vi "Lab Panel V4.89.vi"() -> ()   [LabVIEW 2013] (continued)
                    n844 = stacked-sequence {
                      seq-local: [w1534 _] -> [_ w1538]
                      tunnel: w1532 -> [_ w1548]
                      tunnel: w1531 -> [_ w1547]
                      tunnel: w1530 -> [_ w1546]
                      tunnel: w1529 -> [_ w1545]
                      tunnel: w1528 -> [_ w1544]
                      tunnel: [_ w1543] -> w1527
                      tunnel: w1526 -> [_ w1542]
                      tunnel: w1525 -> [_ w1541]
                      tunnel: w1524 -> [_ w1540]
                      tunnel: w1523 -> [w1533 w1539]
                      tunnel: w1522 -> [_ w1537]
                      frame #0 {
                        n845 = Unbundle(w1533) -> ("AMPS"=w1536:dbl)  [unwired: 4 out]
                        n846 = call "Check For Amps on v1.vi"("ID"="LAB04-1", "amps"=w1536) -> ("amps"=w1534:bool)  [unwired: 9 in]
                      }
                      frame #1 {
                        n847 = case shown="True" w1538 {
                          tunnel: w1548 -> [_ w1561]
                          tunnel: w1547 -> [_ w1560]
                          tunnel: w1546 -> [_ w1559]
                          tunnel: w1545 -> [_ w1558]
                          tunnel: w1544 -> [_ w1557]
                          tunnel: [errorcluster {"status"=FALSE, "code"=0, "source"=""} ("error out") w1556] -> w1543
                          tunnel: w1542 -> [_ w1555]
                          tunnel: w1541 -> [_ w1554]
                          tunnel: w1540 -> [_ w1553]
                          tunnel: w1539 -> [_ w1552]
                          tunnel: w1537 -> [_ w1551]
                          frame False {
                            w1549 = FALSE
                            n848 = local write "RUN LAB04-1"(w1549) -> ()
                            n849 = local write "run lab04-1"(w1549) -> ()
                          }
                          frame True {
                            n850 = stacked-sequence {
                              seq-local: [w1562 _ _ _ _] -> [_ w1586 _ _ _]
                              tunnel: w1561 -> [w1567 _ _ _ _]
                              tunnel: w1560 -> [w1563 _ _ _ _]
                              tunnel: w1559 -> [w1577 _ _ _ _]
                              tunnel: w1558 -> [w1570 _ _ _ _]
                              tunnel: w1557 -> [w1565 _ _ _ _]
                              tunnel: [_ w1581 _ _ _] -> w1556
                              tunnel: w1555 -> [_ _ _ w1607 _]
                              tunnel: w1554 -> [_ _ _ w1606 _]
                              tunnel: w1553 -> [_ _ _ w1605 _]
                              tunnel: w1552 -> [_ _ _ _ _]
                              tunnel: w1551 -> [_ _ _ _ w1621]
                              frame #0 {
                                w1564 = "\\"
                                n851 = local read "SET LAB04-1"() -> (w1572:T5)
                                n852 = case shown="\"CYCLE TEST\"" w1577 {
                                tunnel: ["L04-1-CHART TEST-" "L04-1-CYCLE TEST-" "L04-1-T-RISE TEST-"] -> w1573
                                frame "CHART TEST", Default {
                                }
                                frame "CYCLE TEST" {
                                }
                                frame "T-RISE TEST" {
                                }
                                }
                                n853 = Unbundle(w1572) -> ("DESCRIPTION"=w1571:string)  [unwired: 4 out]
                                n854 = Concatenate Strings(w1567, "\\", w1565, w1564, w1563, w1564) -> (w1574:string)
                                n855 = String To Path(string=w1574) -> (path=w1576:path)
                                n856 = Concatenate Strings(w1574, w1573, w1571, "-", w1570, ".tdms") -> (w1562:string)
                                n857 = Create Folder(path (use dialog)=w1576) -> (error out=w1575:errorcluster)  [unwired: 2 in, 2 out]
                                n858 = global write "Global 1.vi" "LAB04-1 FILE"(w1562) -> ()
                                n859 = call <vilib>:"Clear Errors.vi"("error in (no error)"=w1575) -> ()  [unwired: 6 in, 1 out]
                              }
                              frame #1 {
                                (unwired) FALSE
                                n860 = String To Path(string=w1586) -> (path=w1582:path)
                                n861 = TDMS Open(6:FALSE, 10:T20."create or replace" ("operation (0:open)"), 11:w1582) -> (0:w1581:errorcluster, 3:→"TDMS LAB04-1":refnum<k34>)  [unwired: 4 in]
                              }
                              frame #2 {
                                n862 = local read "SET LAB04-1"() -> (w1592:T5)
                                n863 = local read "TDMS LAB04-1"() -> (w1603:refnum<k34>)
                                n864 = Build Array("Testers Name", "Description", "Set Test Cycles", "T-Rise minutes", "T-Rise Deg C") -> (w1593:string[])
                                n865 = Unbundle(w1592) -> ("NAME"=w1591:string, "DESCRIPTION"=w1590:string, "CYCLES"=w1589:dbl, "T-RISE mins"=w1588:dbl, "T-RISE deg C"=w1587:dbl)
                                n866 = Number To Decimal String(number=w1589) -> (decimal integer string=w1602:string)  [unwired: 1 in]
                                n867 = Number To Decimal String(number=w1588) -> (decimal integer string=w1601:string)  [unwired: 1 in]
                                n868 = Number To Decimal String(number=w1587) -> (decimal integer string=w1600:string)  [unwired: 1 in]
                                n869 = Build Array(w1591, w1590, w1602, w1601, w1600) -> (w1599:string[])
                                n870 = TDMS Set Properties(5:w1599, 7:w1593, 11:w1603) -> ()  [unwired: 3 in, 4 out]
                              }
                              frame #3 {
                                n871 = local read "DISP LAB04-1"() -> (w1608:T4)
                                n872 = Concatenate Strings("LAB04-1  ", w1607) -> (w1609:string)
                                n873 = Two Button Dialog(message=w1609, 1:w1605, 2:w1606) -> (T button?=w1611:bool)
                                n874 = case shown="True" w1611 {
                                tunnel: w1608 -> [w1618 w1619]
                                tunnel: [w1618 w1619] -> w1615
                                tunnel: [w1617 w1620] -> w1614
                                tunnel: [w1616 w1620] -> w1613
                                frame False {
                                n875 = Unbundle(w1618) -> ("CYCLE"=w1617:dbl, "MINS"=w1616:dbl)  [unwired: 1 out]
                                }
                                frame True {
                                w1620 = 0.0
                                }
                                }
                                n876 = Bundle(cluster=w1615, "CYCLE"=w1614, "MINS"=w1613, "STATUS"="RUN") -> (w1604:T4)
                                n877 = local write "DISP LAB04-1"(w1604) -> ()
                              }
                              frame #4 {
                                n878 = local read "TEMP START LAB04-1"() -> (w1623:cluster{"TL":dbl, "TN":dbl})
                                n879 = Bundle(cluster=w1623, "TL"=w1621, "TN"=w1621) -> (w1622:cluster{"TL":dbl, "TN":dbl})
                                n880 = local write "TEMP START LAB04-1"(w1622) -> ()
                              }
                            }
                          }
                        }
                      }
                    }
                  }
                }
              }
              event "RUN LAB04-2": Value Change {
                n881 = event-data() -> ("NewVal"=w1628:bool)  [unwired: 1 in, 5 out]
                n882 = local write "run lab04-2"(w1628) -> ()
                n883 = case shown="True" w1628 {
                  tunnel: w1634 -> [_ w1672]
                  tunnel: w1633 -> [_ w1671]
                  tunnel: w1631 -> [w1636 w1670]
                  tunnel: w1632 -> [_ w1669]
                  tunnel: w1630 -> [_ w1668]
                  tunnel: [w1635 w1667] -> w1629
                  tunnel: w1627 -> [_ w1666]
                  tunnel: w1626 -> [_ w1665]
                  tunnel: w1625 -> [_ w1664]
                  tunnel: w1624 -> [_ w1662]
                  frame False {
                    # "stop test"
                    n884 = stacked-sequence {
                      tunnel: w1636 -> [w1645 _]
                      tunnel: [w1637 _] -> w1635
                      frame #0 {
                        n885 = local read "DISP LAB04-2"() -> (w1644:T4)
                        n886 = Unbundle(w1644) -> ("CYCLE"=w1642:dbl, "MINS"=w1643:dbl)  [unwired: 1 out]
                        n887 = case shown="\"CYCLE TEST\"" w1645 {
                          tunnel: w1643 -> [_ _ w1652]
                          tunnel: w1642 -> [w1650 w1651 _]
                          tunnel: [w1650 w1651 w1652] -> w1641
                          frame "CHART TEST", Default {
                          }
                          frame "CYCLE TEST" {
                          }
                          frame "T-RISE TEST" {
                          }
                        }
                        n888 = local read "TDMS LAB04-2"() -> (w1649:refnum<k34>)
                        n889 = Build Array("STOPPED") -> (w1646:string[])
                        n890 = Build Array(w1641) -> (w1640:dbl[])
                        n891 = TDMS Write(0:w1649, 5:"TEST RESULT", 7:w1646, 9:w1640) -> (4:w1638:refnum<k34>, 15:w1639:errorcluster)  [unwired: 2 in, 2 out]
                        n892 = TDMS Close(8:w1639, 11:w1638) -> (0:w1637:errorcluster)  [unwired: 1 out]
                      }
                      frame #1 {
                        n893 = local read "DISP LAB04-2"() -> (w1656:T4)
                        n894 = stacked-sequence {
                          tunnel: "LAB04-2" -> [w1658 w1660]
                          frame #0 {
                            n895 = call "sub vi - defrag tdms v1.vi"("panel id"=w1658) -> ("error out"=w1657:errorcluster)  [unwired: 10 in]
                            n896 = local write "data file error"(w1657) -> ()
                          }
                          frame #1 {
                            n897 = call "Save data file (stop) v3.vi"("panel id"=w1660) -> ("network file save error"=w1659:errorcluster)  [unwired: 9 in, 1 out]
                            n898 = local write "RESULT LAB04-2"(FALSE) -> ()
                            n899 = local write "data file error"(w1659) -> ()
                          }
                        }
                        n900 = Bundle(cluster=w1656, "STATUS"="STOP") -> (w1654:T4)  [unwired: 2 in]
                        n901 = local write "DISP LAB04-2"(w1654) -> ()
                      }
                    }
                  }
                  frame True {
                    n902 = local read "SIG LAB04-2"() -> (w1663:T2)
                    n903 = stacked-sequence {
                      seq-local: [w1674 _] -> [_ w1678]
                      tunnel: w1672 -> [_ w1688]
                      tunnel: w1671 -> [_ w1687]
                      tunnel: w1670 -> [_ w1686]
                      tunnel: w1669 -> [_ w1685]
                      tunnel: w1668 -> [_ w1684]
                      tunnel: [_ w1683] -> w1667
                      tunnel: w1666 -> [_ w1682]
                      tunnel: w1665 -> [_ w1681]
                      tunnel: w1664 -> [_ w1680]
                      tunnel: w1663 -> [w1673 w1679]
                      tunnel: w1662 -> [_ w1677]
                      frame #0 {
                        n904 = Unbundle(w1673) -> ("AMPS"=w1676:dbl)  [unwired: 4 out]
                        n905 = call "Check For Amps on v1.vi"("ID"="LAB04-2", "amps"=w1676) -> ("amps"=w1674:bool)  [unwired: 9 in]
                      }
                      frame #1 {
                        n906 = case shown="True" w1678 {
                          tunnel: w1688 -> [_ w1701]
                          tunnel: w1687 -> [_ w1700]
                          tunnel: w1686 -> [_ w1699]
                          tunnel: w1685 -> [_ w1698]
                          tunnel: w1684 -> [_ w1697]
                          tunnel: [errorcluster {"status"=FALSE, "code"=0, "source"=""} ("error out") w1696] -> w1683
                          tunnel: w1682 -> [_ w1695]
                          tunnel: w1681 -> [_ w1694]
                          tunnel: w1680 -> [_ w1693]
                          tunnel: w1679 -> [_ w1692]
                          tunnel: w1677 -> [_ w1691]
                          frame False {
                            w1689 = FALSE
                            n907 = local write "RUN LAB04-2"(w1689) -> ()
                            n908 = local write "run lab04-2"(w1689) -> ()
                          }
                          frame True {
                            n909 = stacked-sequence {
                              seq-local: [w1702 _ _ _ _] -> [_ w1726 _ _ _]
                              tunnel: w1701 -> [w1707 _ _ _ _]
                              tunnel: w1700 -> [w1703 _ _ _ _]
                              tunnel: w1699 -> [w1717 _ _ _ _]
                              tunnel: w1698 -> [w1710 _ _ _ _]
                              tunnel: w1697 -> [w1705 _ _ _ _]
                              tunnel: [_ w1721 _ _ _] -> w1696
                              tunnel: w1695 -> [_ _ _ w1747 _]
                              tunnel: w1694 -> [_ _ _ w1746 _]
                              tunnel: w1693 -> [_ _ _ w1745 _]
                              tunnel: w1692 -> [_ _ _ _ _]
                              tunnel: w1691 -> [_ _ _ _ w1761]
                              frame #0 {
                                w1704 = "\\"
                                n910 = local read "SET LAB04-2"() -> (w1712:T5)
                                n911 = case shown="\"CHART TEST\", Default" w1717 {
                                tunnel: ["L04-2-CHART TEST-" "L04-2-CYCLE TEST-" "L04-2-T-RISE TEST-"] -> w1713
                                frame "CHART TEST", Default {
                                }
                                frame "CYCLE TEST" {
                                }
                                frame "T-RISE TEST" {
                                }
                                }
                                n912 = Unbundle(w1712) -> ("DESCRIPTION"=w1711:string)  [unwired: 4 out]
                                n913 = Concatenate Strings(w1707, "\\", w1705, w1704, w1703, w1704) -> (w1714:string)
                                n914 = String To Path(string=w1714) -> (path=w1716:path)
                                n915 = Concatenate Strings(w1714, w1713, w1711, "-", w1710, ".tdms") -> (w1702:string)
                                n916 = Create Folder(path (use dialog)=w1716) -> (error out=w1715:errorcluster)  [unwired: 2 in, 2 out]
                                n917 = global write "Global 1.vi" "LAB04-2 FILE"(w1702) -> ()
                                n918 = call <vilib>:"Clear Errors.vi"("error in (no error)"=w1715) -> ()  [unwired: 6 in, 1 out]
                              }
                              frame #1 {
                                (unwired) FALSE
                                n919 = String To Path(string=w1726) -> (path=w1722:path)
                                n920 = TDMS Open(6:FALSE, 10:T20."create or replace" ("operation (0:open)"), 11:w1722) -> (0:w1721:errorcluster, 3:→"TDMS LAB04-2":refnum<k34>)  [unwired: 4 in]
                              }
                              frame #2 {
                                n921 = local read "SET LAB04-2"() -> (w1732:T5)
                                n922 = local read "TDMS LAB04-2"() -> (w1743:refnum<k34>)
                                n923 = Build Array("Testers Name", "Description", "Set Test Cycles", "T-Rise minutes", "T-Rise Deg C") -> (w1733:string[])
                                n924 = Unbundle(w1732) -> ("NAME"=w1731:string, "DESCRIPTION"=w1730:string, "CYCLES"=w1729:dbl, "T-RISE mins"=w1728:dbl, "T-RISE deg C"=w1727:dbl)
                                n925 = Number To Decimal String(number=w1729) -> (decimal integer string=w1742:string)  [unwired: 1 in]
                                n926 = Number To Decimal String(number=w1728) -> (decimal integer string=w1741:string)  [unwired: 1 in]
                                n927 = Number To Decimal String(number=w1727) -> (decimal integer string=w1740:string)  [unwired: 1 in]
                                n928 = Build Array(w1731, w1730, w1742, w1741, w1740) -> (w1739:string[])
                                n929 = TDMS Set Properties(5:w1739, 7:w1733, 11:w1743) -> ()  [unwired: 3 in, 4 out]
                              }
                              frame #3 {
                                n930 = local read "DISP LAB04-2"() -> (w1748:T4)
                                n931 = Concatenate Strings("LAB04-2 ", w1747) -> (w1749:string)
                                n932 = Two Button Dialog(message=w1749, 1:w1745, 2:w1746) -> (T button?=w1751:bool)
                                n933 = case shown="True" w1751 {
                                tunnel: w1748 -> [w1758 w1759]
                                tunnel: [w1758 w1759] -> w1755
                                tunnel: [w1757 w1760] -> w1754
                                tunnel: [w1756 w1760] -> w1753
                                frame False {
                                n934 = Unbundle(w1758) -> ("CYCLE"=w1757:dbl, "MINS"=w1756:dbl)  [unwired: 1 out]
                                }
                                frame True {
                                w1760 = 0.0
                                }
                                }
                                n935 = Bundle(cluster=w1755, "CYCLE"=w1754, "MINS"=w1753, "STATUS"="RUN") -> (w1744:T4)
                                n936 = local write "DISP LAB04-2"(w1744) -> ()
                              }
                              frame #4 {
                                n937 = local read "TEMP START LAB04-2"() -> (w1763:cluster{"TL":dbl, "TN":dbl})
                                n938 = Bundle(cluster=w1763, "TL"=w1761, "TN"=w1761) -> (w1762:cluster{"TL":dbl, "TN":dbl})
                                n939 = local write "TEMP START LAB04-2"(w1762) -> ()
                              }
                            }
                          }
                        }
                      }
                    }
                  }
                }
              }
              event "RUN LAB05-1": Value Change {
                n940 = event-data() -> ("NewVal"=w1768:bool)  [unwired: 1 in, 5 out]
                n941 = local write "run lab05-1"(w1768) -> ()
                n942 = case shown="True" w1768 {
                  tunnel: w1774 -> [_ w1812]
                  tunnel: w1773 -> [_ w1811]
                  tunnel: w1771 -> [w1776 w1810]
                  tunnel: w1772 -> [_ w1809]
                  tunnel: w1770 -> [_ w1808]
                  tunnel: [w1775 w1807] -> w1769
                  tunnel: w1767 -> [_ w1806]
                  tunnel: w1766 -> [_ w1805]
                  tunnel: w1765 -> [_ w1804]
                  tunnel: w1764 -> [_ w1802]
                  frame False {
                    # "stop test"
                    n943 = stacked-sequence {
                      tunnel: w1776 -> [w1785 _]
                      tunnel: [w1777 _] -> w1775
                      frame #0 {
                        n944 = local read "DISP LAB05-1"() -> (w1784:T4)
                        n945 = Unbundle(w1784) -> ("CYCLE"=w1782:dbl, "MINS"=w1783:dbl)  [unwired: 1 out]
                        n946 = case shown="\"CYCLE TEST\"" w1785 {
                          tunnel: w1783 -> [_ _ w1792]
                          tunnel: w1782 -> [w1790 w1791 _]
                          tunnel: [w1790 w1791 w1792] -> w1781
                          frame "CHART TEST", Default {
                          }
                          frame "CYCLE TEST" {
                          }
                          frame "T-RISE TEST" {
                          }
                        }
                        n947 = local read "TDMS LAB05-1"() -> (w1789:refnum<k34>)
                        n948 = Build Array("STOPPED") -> (w1786:string[])
                        n949 = Build Array(w1781) -> (w1780:dbl[])
                        n950 = TDMS Write(0:w1789, 5:"TEST RESULT", 7:w1786, 9:w1780) -> (4:w1778:refnum<k34>, 15:w1779:errorcluster)  [unwired: 2 in, 2 out]
                        n951 = TDMS Close(8:w1779, 11:w1778) -> (0:w1777:errorcluster)  [unwired: 1 out]
                      }
                      frame #1 {
                        n952 = local read "DISP LAB05-1"() -> (w1796:T4)
                        n953 = stacked-sequence {
                          tunnel: "LAB05-1" -> [w1798 w1800]
                          frame #0 {
                            n954 = call "sub vi - defrag tdms v1.vi"("panel id"=w1798) -> ("error out"=w1797:errorcluster)  [unwired: 10 in]
                            n955 = local write "data file error"(w1797) -> ()
                          }
                          frame #1 {
                            n956 = call "Save data file (stop) v3.vi"("panel id"=w1800) -> ("network file save error"=w1799:errorcluster)  [unwired: 9 in, 1 out]
                            n957 = local write "RESULT LAB05-1"(FALSE) -> ()
                            n958 = local write "data file error"(w1799) -> ()
                          }
                        }
                        n959 = Bundle(cluster=w1796, "STATUS"="STOP") -> (w1794:T4)  [unwired: 2 in]
                        n960 = local write "DISP LAB05-1"(w1794) -> ()
                      }
                    }
                  }
                  frame True {
                    n961 = local read "SIG LAB05-1"() -> (w1803:T2)
                    n962 = stacked-sequence {
                      seq-local: [w1814 _] -> [_ w1818]
                      tunnel: w1812 -> [_ w1828]
                      tunnel: w1811 -> [_ w1827]
                      tunnel: w1810 -> [_ w1826]
                      tunnel: w1809 -> [_ w1825]
                      tunnel: w1808 -> [_ w1824]
                      tunnel: [_ w1823] -> w1807
                      tunnel: w1806 -> [_ w1822]
                      tunnel: w1805 -> [_ w1821]
                      tunnel: w1804 -> [_ w1820]
                      tunnel: w1803 -> [w1813 w1819]
                      tunnel: w1802 -> [_ w1817]
                      frame #0 {
                        n963 = Unbundle(w1813) -> ("AMPS"=w1816:dbl)  [unwired: 4 out]
                        n964 = call "Check For Amps on v1.vi"("ID"="LAB05-1", "amps"=w1816) -> ("amps"=w1814:bool)  [unwired: 9 in]
                      }
                      frame #1 {
                        n965 = case shown="True" w1818 {
                          tunnel: w1828 -> [_ w1841]
                          tunnel: w1827 -> [_ w1840]
                          tunnel: w1826 -> [_ w1839]
                          tunnel: w1825 -> [_ w1838]
                          tunnel: w1824 -> [_ w1837]
                          tunnel: [errorcluster {"status"=FALSE, "code"=0, "source"=""} ("error out") w1836] -> w1823
                          tunnel: w1822 -> [_ w1835]
                          tunnel: w1821 -> [_ w1834]
                          tunnel: w1820 -> [_ w1833]
                          tunnel: w1819 -> [_ w1832]
                          tunnel: w1817 -> [_ w1831]
                          frame False {
                            w1829 = FALSE
                            n966 = local write "RUN LAB05-1"(w1829) -> ()
                            n967 = local write "run lab05-1"(w1829) -> ()
                          }
                          frame True {
                            n968 = stacked-sequence {
                              seq-local: [w1842 _ _ _ _] -> [_ w1866 _ _ _]
                              tunnel: w1841 -> [w1847 _ _ _ _]
                              tunnel: w1840 -> [w1843 _ _ _ _]
                              tunnel: w1839 -> [w1857 _ _ _ _]
                              tunnel: w1838 -> [w1850 _ _ _ _]
                              tunnel: w1837 -> [w1845 _ _ _ _]
                              tunnel: [_ w1861 _ _ _] -> w1836
                              tunnel: w1835 -> [_ _ _ w1886 _]
                              tunnel: w1834 -> [_ _ _ w1885 _]
                              tunnel: w1833 -> [_ _ _ w1884 _]
                              tunnel: w1832 -> [_ _ _ _ _]
                              tunnel: w1831 -> [_ _ _ _ w1901]
                              frame #0 {
                                w1844 = "\\"
                                n969 = local read "SET LAB05-1"() -> (w1852:T5)
                                n970 = case shown="\"CYCLE TEST\"" w1857 {
                                tunnel: ["L05-1-CHART TEST-" "L05-1-CYCLE TEST-" "L05-1-T-RISE TEST-"] -> w1853
                                frame "CHART TEST", Default {
                                }
                                frame "CYCLE TEST" {
                                }
                                frame "T-RISE TEST" {
                                }
                                }
                                n971 = Unbundle(w1852) -> ("DESCRIPTION"=w1851:string)  [unwired: 4 out]
                                n972 = Concatenate Strings(w1847, "\\", w1845, w1844, w1843, w1844) -> (w1854:string)
                                n973 = String To Path(string=w1854) -> (path=w1856:path)
                                n974 = Concatenate Strings(w1854, w1853, w1851, "-", w1850, ".tdms") -> (w1842:string)
                                n975 = Create Folder(path (use dialog)=w1856) -> (error out=w1855:errorcluster)  [unwired: 2 in, 2 out]
                                n976 = global write "Global 1.vi" "LAB05-1 FILE"(w1842) -> ()
                                n977 = call <vilib>:"Clear Errors.vi"("error in (no error)"=w1855) -> ()  [unwired: 6 in, 1 out]
                              }
                              frame #1 {
                                (unwired) FALSE
                                n978 = String To Path(string=w1866) -> (path=w1862:path)
                                n979 = TDMS Open(6:FALSE, 10:T20."create or replace" ("operation (0:open)"), 11:w1862) -> (0:w1861:errorcluster, 3:→"TDMS LAB05-1":refnum<k34>)  [unwired: 4 in]
                              }
                              frame #2 {
                                n980 = local read "SET LAB05-1"() -> (w1872:T5)
                                n981 = local read "TDMS LAB05-1"() -> (w1883:refnum<k34>)
                                n982 = Build Array("Testers Name", "Description", "Set Test Cycles", "T-Rise minutes", "T-Rise Deg C") -> (w1873:string[])
                                n983 = Unbundle(w1872) -> ("NAME"=w1871:string, "DESCRIPTION"=w1870:string, "CYCLES"=w1869:dbl, "T-RISE mins"=w1868:dbl, "T-RISE deg C"=w1867:dbl)
                                n984 = Number To Decimal String(number=w1869) -> (decimal integer string=w1882:string)  [unwired: 1 in]
                                n985 = Number To Decimal String(number=w1868) -> (decimal integer string=w1881:string)  [unwired: 1 in]
                                n986 = Number To Decimal String(number=w1867) -> (decimal integer string=w1880:string)  [unwired: 1 in]
                                n987 = Build Array(w1871, w1870, w1882, w1881, w1880) -> (w1879:string[])
                                n988 = TDMS Set Properties(5:w1879, 7:w1873, 11:w1883) -> ()  [unwired: 3 in, 4 out]
                              }
                              frame #3 {
                                n989 = local read "DISP LAB05-1"() -> (w1888:T4)
                                n990 = Concatenate Strings("LAB05-1  ", w1886) -> (w1889:string)
                                n991 = Two Button Dialog(message=w1889, 1:w1884, 2:w1885) -> (T button?=w1891:bool)
                                n992 = case shown="True" w1891 {
                                tunnel: w1888 -> [w1898 w1899]
                                tunnel: [w1898 w1899] -> w1895
                                tunnel: [w1897 w1900] -> w1894
                                tunnel: [w1896 w1900] -> w1893
                                frame False {
                                n993 = Unbundle(w1898) -> ("CYCLE"=w1897:dbl, "MINS"=w1896:dbl)  [unwired: 1 out]
                                }
                                frame True {
                                w1900 = 0.0
                                }
                                }
                                n994 = Bundle(cluster=w1895, "CYCLE"=w1894, "MINS"=w1893, "STATUS"="RUN") -> (w1887:T4)
                                n995 = local write "DISP LAB05-1"(w1887) -> ()
                              }
                              frame #4 {
                                n996 = local read "TEMP START LAB05-1"() -> (w1903:cluster{"TL":dbl, "TN":dbl})
                                n997 = Bundle(cluster=w1903, "TL"=w1901, "TN"=w1901) -> (w1902:cluster{"TL":dbl, "TN":dbl})
                                n998 = local write "TEMP START LAB05-1"(w1902) -> ()
                              }
                            }
                          }
                        }
                      }
                    }
                  }
                }
              }
              event "RUN LAB05-2": Value Change {
                n999 = event-data() -> ("NewVal"=w1909:bool)  [unwired: 1 in, 5 out]
                n1000 = local read "SIG LAB05-2"() -> (w1905:T2)
                n1001 = case shown="True" w1909 {
                  tunnel: w1915 -> [_ w1953]
                  tunnel: w1914 -> [_ w1952]
                  tunnel: w1912 -> [w1917 w1951]
                  tunnel: w1913 -> [_ w1950]
                  tunnel: w1911 -> [_ w1949]
                  tunnel: [w1916 w1948] -> w1910
                  tunnel: w1908 -> [_ w1947]
                  tunnel: w1907 -> [_ w1946]
                  tunnel: w1906 -> [_ w1945]
                  tunnel: w1905 -> [_ w1944]
                  tunnel: w1904 -> [_ w1943]
                  frame False {
                    # "stop test"
                    n1002 = stacked-sequence {
                      tunnel: w1917 -> [w1926 _]
                      tunnel: [w1918 _] -> w1916
                      frame #0 {
                        n1003 = local read "DISP LAB05-2"() -> (w1925:T4)
                        n1004 = Unbundle(w1925) -> ("CYCLE"=w1923:dbl, "MINS"=w1924:dbl)  [unwired: 1 out]
                        n1005 = case shown="\"CYCLE TEST\"" w1926 {
                          tunnel: w1924 -> [_ _ w1933]
                          tunnel: w1923 -> [w1931 w1932 _]
                          tunnel: [w1931 w1932 w1933] -> w1922
                          frame "CHART TEST", Default {
                          }
                          frame "CYCLE TEST" {
                          }
                          frame "T-RISE TEST" {
                          }
                        }
                        n1006 = local read "TDMS LAB05-2"() -> (w1930:refnum<k34>)
                        n1007 = Build Array("STOPPED") -> (w1927:string[])
                        n1008 = Build Array(w1922) -> (w1921:dbl[])
                        n1009 = TDMS Write(0:w1930, 5:"TEST RESULT", 7:w1927, 9:w1921) -> (4:w1919:refnum<k34>, 15:w1920:errorcluster)  [unwired: 2 in, 2 out]
                        n1010 = TDMS Close(8:w1920, 11:w1919) -> (0:w1918:errorcluster)  [unwired: 1 out]
                      }
                      frame #1 {
                        n1011 = local read "DISP LAB05-2"() -> (w1937:T4)
                        n1012 = stacked-sequence {
                          tunnel: "LAB05-2" -> [w1939 w1941]
                          frame #0 {
                            n1013 = call "sub vi - defrag tdms v1.vi"("panel id"=w1939) -> ("error out"=w1938:errorcluster)  [unwired: 10 in]
                            n1014 = local write "data file error"(w1938) -> ()
                          }
                          frame #1 {
                            n1015 = local write "RESULT LAB05-2"(FALSE) -> ()
                            n1016 = call "Save data file (stop) v3.vi"("panel id"=w1941) -> ("network file save error"=w1940:errorcluster)  [unwired: 9 in, 1 out]
                            n1017 = local write "data file error"(w1940) -> ()
                          }
                        }
                        n1018 = Bundle(cluster=w1937, "STATUS"="STOP") -> (w1935:T4)  [unwired: 2 in]
                        n1019 = local write "DISP LAB05-2"(w1935) -> ()
                      }
                    }
                  }
                  frame True {
                    n1020 = stacked-sequence {
                      seq-local: [w1955 _] -> [_ w1959]
                      tunnel: w1953 -> [_ w1969]
                      tunnel: w1952 -> [_ w1968]
                      tunnel: w1951 -> [_ w1967]
                      tunnel: w1950 -> [_ w1966]
                      tunnel: w1949 -> [_ w1965]
                      tunnel: [_ w1964] -> w1948
                      tunnel: w1947 -> [_ w1963]
                      tunnel: w1946 -> [_ w1962]
                      tunnel: w1945 -> [_ w1961]
                      tunnel: w1944 -> [w1954 w1960]
                      tunnel: w1943 -> [_ w1958]
                      frame #0 {
                        n1021 = Unbundle(w1954) -> ("AMPS"=w1957:dbl)  [unwired: 4 out]
                        n1022 = call "Check For Amps on v1.vi"("ID"="LAB05-2", "amps"=w1957) -> ("amps"=w1955:bool)  [unwired: 9 in]
                      }
                      frame #1 {
                        n1023 = case shown="True" w1959 {
                          tunnel: w1969 -> [_ w1982]
                          tunnel: w1968 -> [_ w1981]
                          tunnel: w1967 -> [_ w1980]
                          tunnel: w1966 -> [_ w1979]
                          tunnel: w1965 -> [_ w1978]
                          tunnel: [errorcluster {"status"=FALSE, "code"=0, "source"=""} ("error out") w1977] -> w1964
                          tunnel: w1963 -> [_ w1976]
                          tunnel: w1962 -> [_ w1975]
                          tunnel: w1961 -> [_ w1974]
                          tunnel: w1960 -> [_ w1973]
                          tunnel: w1958 -> [_ w1972]
                          frame False {
                            w1970 = FALSE
                            n1024 = local write "RUN LAB05-2"(w1970) -> ()
                            n1025 = local write "run lab05-2"(w1970) -> ()
                          }
                          frame True {
                            n1026 = stacked-sequence {
                              seq-local: [w1983 _ _ _ _] -> [_ w2007 _ _ _]
                              tunnel: w1982 -> [w1988 _ _ _ _]
                              tunnel: w1981 -> [w1984 _ _ _ _]
                              tunnel: w1980 -> [w1998 _ _ _ _]
                              tunnel: w1979 -> [w1991 _ _ _ _]
                              tunnel: w1978 -> [w1986 _ _ _ _]
                              tunnel: [_ w2002 _ _ _] -> w1977
                              tunnel: w1976 -> [_ _ _ w2027 _]
                              tunnel: w1975 -> [_ _ _ w2026 _]
                              tunnel: w1974 -> [_ _ _ w2025 _]
                              tunnel: w1973 -> [_ _ _ _ _]
                              tunnel: w1972 -> [_ _ _ _ w2042]
                              frame #0 {
                                w1985 = "\\"
                                n1027 = local read "SET LAB05-2"() -> (w1993:T5)
                                n1028 = case shown="\"CYCLE TEST\"" w1998 {
                                tunnel: ["L05-2-CHART TEST-" "L05-2-CYCLE TEST-" "L05-2-T-RISE TEST-"] -> w1994
                                frame "CHART TEST", Default {
                                }
                                frame "CYCLE TEST" {
                                }
                                frame "T-RISE TEST" {
                                }
                                }
                                n1029 = Unbundle(w1993) -> ("DESCRIPTION"=w1992:string)  [unwired: 4 out]
                                n1030 = Concatenate Strings(w1988, "\\", w1986, w1985, w1984, w1985) -> (w1995:string)
                                n1031 = String To Path(string=w1995) -> (path=w1997:path)
                                n1032 = Concatenate Strings(w1995, w1994, w1992, "-", w1991, ".tdms") -> (w1983:string)
                                n1033 = Create Folder(path (use dialog)=w1997) -> (error out=w1996:errorcluster)  [unwired: 2 in, 2 out]
                                n1034 = global write "Global 1.vi" "LAB05-2 FILE"(w1983) -> ()
                                n1035 = call <vilib>:"Clear Errors.vi"("error in (no error)"=w1996) -> ()  [unwired: 6 in, 1 out]
                              }
                              frame #1 {
                                (unwired) FALSE
                                n1036 = String To Path(string=w2007) -> (path=w2003:path)
                                n1037 = TDMS Open(6:FALSE, 10:T20."create or replace" ("operation (0:open)"), 11:w2003) -> (0:w2002:errorcluster, 3:→"TDMS LAB05-2":refnum<k34>)  [unwired: 4 in]
                              }
                              frame #2 {
                                n1038 = local read "SET LAB05-2"() -> (w2013:T5)
                                n1039 = local read "TDMS LAB05-2"() -> (w2024:refnum<k34>)
                                n1040 = Build Array("Testers Name", "Description", "Set Test Cycles", "T-Rise minutes", "T-Rise Deg C") -> (w2014:string[])
                                n1041 = Unbundle(w2013) -> ("NAME"=w2012:string, "DESCRIPTION"=w2011:string, "CYCLES"=w2010:dbl, "T-RISE mins"=w2009:dbl, "T-RISE deg C"=w2008:dbl)
                                n1042 = Number To Decimal String(number=w2010) -> (decimal integer string=w2023:string)  [unwired: 1 in]
                                n1043 = Number To Decimal String(number=w2009) -> (decimal integer string=w2022:string)  [unwired: 1 in]
                                n1044 = Number To Decimal String(number=w2008) -> (decimal integer string=w2021:string)  [unwired: 1 in]
                                n1045 = Build Array(w2012, w2011, w2023, w2022, w2021) -> (w2020:string[])
                                n1046 = TDMS Set Properties(5:w2020, 7:w2014, 11:w2024) -> ()  [unwired: 3 in, 4 out]
                              }
                              frame #3 {
                                n1047 = local read "DISP LAB05-2"() -> (w2029:T4)
                                n1048 = Concatenate Strings("LAB05-2  ", w2027) -> (w2030:string)
                                n1049 = Two Button Dialog(message=w2030, 1:w2025, 2:w2026) -> (T button?=w2032:bool)
                                n1050 = case shown="True" w2032 {
                                tunnel: w2029 -> [w2039 w2040]
                                tunnel: [w2039 w2040] -> w2036
                                tunnel: [w2038 w2041] -> w2035
                                tunnel: [w2037 w2041] -> w2034
                                frame False {
                                n1051 = Unbundle(w2039) -> ("CYCLE"=w2038:dbl, "MINS"=w2037:dbl)  [unwired: 1 out]
                                }
                                frame True {
                                w2041 = 0.0
                                }
                                }
                                n1052 = Bundle(cluster=w2036, "CYCLE"=w2035, "MINS"=w2034, "STATUS"="RUN") -> (w2028:T4)
                                n1053 = local write "DISP LAB05-2"(w2028) -> ()
                              }
                              frame #4 {
                                n1054 = local read "TEMP START LAB05-2"() -> (w2044:cluster{"TL":dbl, "TN":dbl})
                                n1055 = Bundle(cluster=w2044, "TL"=w2042, "TN"=w2042) -> (w2043:cluster{"TL":dbl, "TN":dbl})
                                n1056 = local write "TEMP START LAB05-2"(w2043) -> ()
                              }
                            }
                          }
                        }
                      }
                    }
                  }
                }
                n1057 = local write "run lab05-2"(w1909) -> ()
              }
            }
            n1058 = local write "data file error"(w613) -> ()
          }
          frame #4 {
            # "check if test cycles reached for cycle tests, if so then test pass"
            n1059 = stacked-sequence {
              tunnel: w2064 -> [_ _ _ _ _ _ _ _ _ _]
              tunnel: w2063 -> [_ _ _ _ _ _ _ _ _ _]
              tunnel: w2062 -> [_ _ _ _ _ _ _ _ _ _]
              tunnel: w2061 -> [_ _ _ _ _ _ _ _ _ _]
              tunnel: w2060 -> [_ _ _ _ _ _ _ _ _ _]
              tunnel: w2059 -> [_ _ _ _ _ _ _ _ _ _]
              tunnel: w2058 -> [_ _ _ _ _ _ _ _ _ _]
              tunnel: w2057 -> [_ _ _ _ _ _ _ _ _ _]
              tunnel: w2056 -> [_ _ _ _ _ _ _ _ _ _]
              tunnel: w2055 -> [_ _ _ _ _ _ _ _ _ _]
              tunnel: w2054 -> [w2070 _ _ _ _ _ _ _ _ _]
              tunnel: w2053 -> [_ w2105 _ _ _ _ _ _ _ _]
              tunnel: w2052 -> [_ _ w2145 _ _ _ _ _ _ _]
              tunnel: w2051 -> [_ _ _ w2185 _ _ _ _ _ _]
              tunnel: w2050 -> [_ _ _ _ w2225 _ _ _ _ _]
              tunnel: w2049 -> [_ _ _ _ _ w2265 _ _ _ _]
              tunnel: w2048 -> [_ _ _ _ _ _ w2305 _ _ _]
              tunnel: w2047 -> [_ _ _ _ _ _ _ w2345 _ _]
              tunnel: w2046 -> [_ _ _ _ _ _ _ _ w2385 _]
              tunnel: w2045 -> [_ _ _ _ _ _ _ _ _ w2425]
              frame #0 {
                # "LAB01-1"
                n1060 = Less?(x=w2070, y=2) -> (x < y?=w2068:bool)
                n1061 = local read "DISP LAB01-1"() -> (w2071:T4)
                n1062 = Unbundle(w2071) -> ("STATUS"=w2065:string)  [unwired: 2 out]
                n1063 = Equal?(x=w2065, y="RUN") -> (x = y?=w2067:bool)
                n1064 = And(x=w2067, y=w2068) -> (x .and. y?=w2066:bool)
                n1065 = case shown="True" w2066 {
                  tunnel: w2071 -> [_ w2076]
                  tunnel: w2070 -> [_ w2080]
                  frame False {
                  }
                  frame True {
                    n1066 = local read "SET LAB01-1"() -> (w2082:T5)
                    n1067 = local read "TDMS LAB01-1"() -> (w2075:refnum<k34>)
                    n1068 = Unbundle(w2082) -> ("CYCLES"=w2073:dbl, "T-RISE mins"=w2079:dbl)  [unwired: 3 out]
                    n1069 = case shown="\"CYCLE TEST\"" w2080 {
                      tunnel: w2079 -> [_ _ w2089]
                      tunnel: [w2084 w2086 w2089] -> w2078
                      tunnel: w2073 -> [w2084 w2086 _]
                      tunnel: ["CHART PASS" "CYCLE PASS" "T-RISE PASS"] -> w2077
                      frame "CHART TEST", Default {
                      }
                      frame "CYCLE TEST" {
                      }
                      frame "T-RISE TEST" {
                      }
                    }
                    n1070 = Unbundle(w2076) -> ("CYCLE"=w2081:dbl)  [unwired: 2 out]
                    n1071 = Increment(x=w2073) -> (x+1=w2074:dbl)
                    n1072 = Greater Or Equal?(x=w2081, y=w2074) -> (x >= y?=w2083:bool)
                    n1073 = case shown="True" w2083 {
                      tunnel: w2078 -> [w2093 _]
                      tunnel: w2077 -> [w2092 _]
                      tunnel: w2076 -> [w2091 _]
                      tunnel: w2075 -> [w2090 _]
                      frame True {
                        n1074 = stacked-sequence {
                          tunnel: w2093 -> [w2097 _]
                          tunnel: w2092 -> [w2095 w2101]
                          tunnel: w2091 -> [_ w2104]
                          tunnel: w2090 -> [w2094 _]
                          frame #0 {
                            n1075 = Build Array(w2095) -> (w2098:string[])
                            n1076 = Build Array(w2097) -> (w2096:dbl[])
                            n1077 = TDMS Write(0:w2094, 5:"TEST PASS", 7:w2098, 9:w2096) -> (15:w2100:errorcluster)  [unwired: 2 in, 3 out]
                            n1078 = local write "data file error"(w2100) -> ()
                          }
                          frame #1 {
                            n1079 = Bundle(cluster=w2104, "STATUS"=w2101) -> (w2102:T4)  [unwired: 2 in]
                            n1080 = local write "RESULT LAB01-1"(TRUE) -> ()
                            n1081 = local write "DISP LAB01-1"(w2102) -> ()
                          }
                        }
                      }
                      frame False {
                      }
                    }
                  }
                }
              }
              frame #1 {
                # "LAB01-2"
                n1082 = Less?(x=w2105, y=2) -> (x < y?=w2108:bool)
                n1083 = local read "DISP LAB01-2"() -> (w2110:T4)
                n1084 = Unbundle(w2110) -> ("STATUS"=w2111:string)  [unwired: 2 out]
                n1085 = Equal?(x=w2111, y="RUN") -> (x = y?=w2107:bool)
                n1086 = And(x=w2107, y=w2108) -> (x .and. y?=w2106:bool)
                n1087 = case shown="True" w2106 {
                  tunnel: w2110 -> [_ w2116]
                  tunnel: w2105 -> [_ w2120]
                  frame False {
                  }
                  frame True {
                    n1088 = local read "SET LAB01-2"() -> (w2122:T5)
                    n1089 = local read "TDMS LAB01-2"() -> (w2115:refnum<k34>)
                    n1090 = Unbundle(w2122) -> ("CYCLES"=w2113:dbl, "T-RISE mins"=w2119:dbl)  [unwired: 3 out]
                    n1091 = case shown="\"T-RISE TEST\"" w2120 {
                      tunnel: w2119 -> [_ _ w2129]
                      tunnel: [w2124 w2126 w2129] -> w2118
                      tunnel: w2113 -> [w2124 w2126 _]
                      tunnel: ["CHART PASS" "CYCLE PASS" "T-RISE PASS"] -> w2117
                      frame "CHART TEST", Default {
                      }
                      frame "CYCLE TEST" {
                      }
                      frame "T-RISE TEST" {
                      }
                    }
                    n1092 = Unbundle(w2116) -> ("CYCLE"=w2121:dbl)  [unwired: 2 out]
                    n1093 = Increment(x=w2113) -> (x+1=w2114:dbl)
                    n1094 = Greater Or Equal?(x=w2121, y=w2114) -> (x >= y?=w2123:bool)
                    n1095 = case shown="True" w2123 {
                      tunnel: w2118 -> [w2133 _]
                      tunnel: w2117 -> [w2132 _]
                      tunnel: w2116 -> [w2131 _]
                      tunnel: w2115 -> [w2130 _]
                      frame True {
                        n1096 = stacked-sequence {
                          tunnel: w2133 -> [w2137 _]
                          tunnel: w2132 -> [w2135 w2141]
                          tunnel: w2131 -> [_ w2144]
                          tunnel: w2130 -> [w2134 _]
                          frame #0 {
                            n1097 = Build Array(w2135) -> (w2138:string[])
                            n1098 = Build Array(w2137) -> (w2136:dbl[])
                            n1099 = TDMS Write(0:w2134, 5:"TEST PASS", 7:w2138, 9:w2136) -> (15:w2140:errorcluster)  [unwired: 2 in, 3 out]
                            n1100 = local write "data file error"(w2140) -> ()
                          }
                          frame #1 {
                            n1101 = Bundle(cluster=w2144, "STATUS"=w2141) -> (w2142:T4)  [unwired: 2 in]
                            n1102 = local write "RESULT LAB01-2"(TRUE) -> ()
                            n1103 = local write "DISP LAB01-2"(w2142) -> ()
                          }
                        }
                      }
                      frame False {
                      }
                    }
                  }
                }
              }
              frame #2 {
                # "LAB02-1"
                n1104 = Less?(x=w2145, y=2) -> (x < y?=w2148:bool)
                n1105 = local read "DISP LAB02-1"() -> (w2150:T4)
                n1106 = Unbundle(w2150) -> ("STATUS"=w2151:string)  [unwired: 2 out]
                n1107 = Equal?(x=w2151, y="RUN") -> (x = y?=w2147:bool)
                n1108 = And(x=w2147, y=w2148) -> (x .and. y?=w2146:bool)
                n1109 = case shown="True" w2146 {
                  tunnel: w2150 -> [_ w2156]
                  tunnel: w2145 -> [_ w2160]
                  frame False {
                  }
                  frame True {
                    n1110 = local read "SET LAB02-1"() -> (w2162:T5)
                    n1111 = local read "TDMS LAB02-1"() -> (w2155:refnum<k34>)
                    n1112 = Unbundle(w2156) -> ("CYCLE"=w2161:dbl)  [unwired: 2 out]
                    n1113 = Unbundle(w2162) -> ("CYCLES"=w2153:dbl, "T-RISE mins"=w2159:dbl)  [unwired: 3 out]
                    n1114 = case shown="\"T-RISE TEST\"" w2160 {
                      tunnel: w2159 -> [_ _ w2169]
                      tunnel: [w2164 w2166 w2169] -> w2158
                      tunnel: w2153 -> [w2164 w2166 _]
                      tunnel: ["CHART PASS" "CYCLE PASS" "T-RISE PASS"] -> w2157
                      frame "CHART TEST", Default {
                      }
                      frame "CYCLE TEST" {
                      }
                      frame "T-RISE TEST" {
                      }
                    }
                    n1115 = Increment(x=w2153) -> (x+1=w2154:dbl)
